vi "Setup.vi"(0 "SettingsFile in":refnum<class "SettingsFile.lvclass">, 1 "ProjectName":string, 2 "FileName":string, 3 "MD5 (optional)":string, 4 "Path":path, 5 "error in (no error)":errorcluster) -> (14 "SettingsFile out":refnum<class "SettingsFile.lvclass">, 19 "error out":errorcluster)   [LabVIEW 2018, in "feGEM DataPacker.lvlib" / "SettingsFile.lvclass"]
uses:
  SettingsFile.lvclass
  SettingsFile.lvclass/SettingsFile.ctl
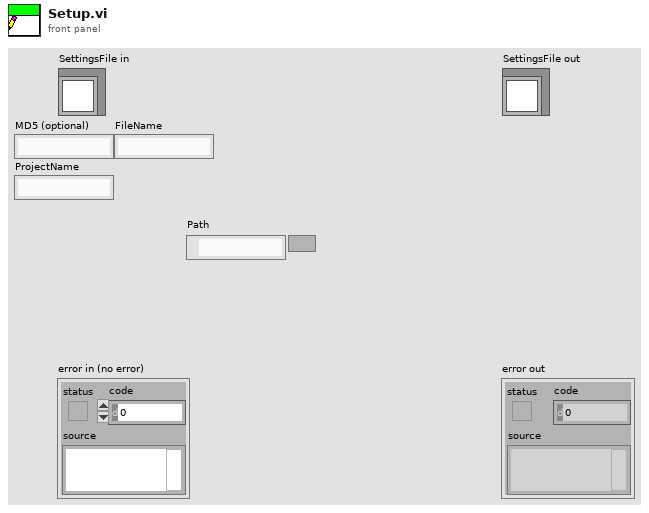
[diagram p1: front panel]
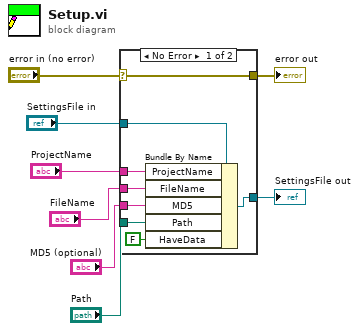
[diagram p0: block diagram]
diagram:
  n1 = case shown="No Error" "error in (no error)" {
    selector: "error in (no error)" -> [w16 w17]
    tunnel: [w16 w17] -> w7
    tunnel: [w14 w18] -> w5
    tunnel: "SettingsFile in" -> [w15 w18]
    tunnel: "Path" -> [w13 _]
    tunnel: "ProjectName" -> [w12 _]
    tunnel: "FileName" -> [w11 _]
    tunnel: "MD5 (optional)" -> [w10 _]
    frame No Error {
      n2 = Bundle By Name(cluster=w15, "ProjectName"=w12, "FileName"=w11, "MD5"=w10, "Path"=w13, "HaveData"=FALSE) -> (w14:refnum<class "SettingsFile.lvclass">)
    }
    frame Error {
    }
  }
  "error out" <- w7
  "SettingsFile out" <- w5
